vi "niFpgaFFTStreamingOutputControlUnit.vi"(0 "reset":bool, 5 "ready for output":bool, 7 "current status":enum8{"idle", "output"}(ring), 9 "execution constants":cluster{"bitmask":u16, "K-16":i8}={"bitmask"=2047, "K-16"=-5}) -> (4 "output valid (inside)":bool, 6 "next status":enum8{"idle", "output"}(ring), 8 "data index":u16, 10 "use buffer 0":bool, 13 "read address 1":u16, 14 "read address 0":u16)   [LabVIEW 2017]
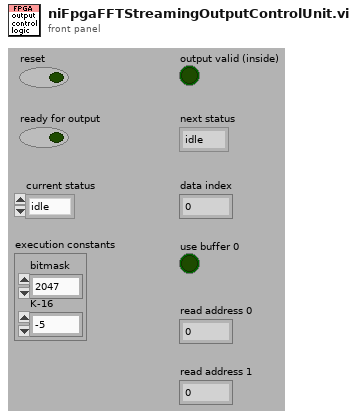
[diagram p1: front panel]
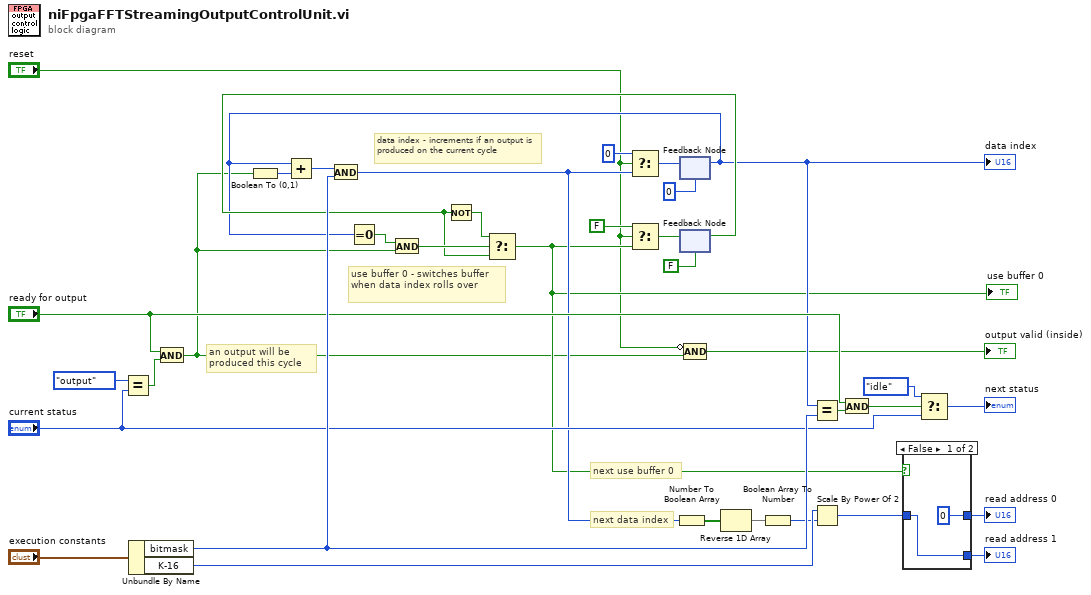
[diagram p0: block diagram]
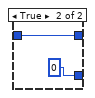
[diagram p2: hidden frame]
diagram:
  # "an output will be produced this cycle"
  # "use buffer 0 - switches buffer when data index rolls over"
  # "data index - increments if an output is produced on the current cycle"
  # "next data index"
  # "next use buffer 0"
  n1 = Equal?(x=enum8{"idle", "output"}."output" ("current status"), y="current status") -> (x = y?=w30:bool)
  n2 = Unbundle By Name("execution constants") -> ("bitmask"=w25:u16, "K-16"=w32:i8)
  n3 = And(x="ready for output", y=w30) -> (x .and. y?=w3:bool)
  n4 = Boolean To (0,1)(Boolean=w3) -> (0, 1=w22:i16)
  n5 = feedback #1(u16 0 ("t")) -> (w7:u16)
  "data index" <- w7
  n6 = Add(x=w7, y=w22) -> (x+y=w21:u16)
  n7 = And(x=w21, y=w25) -> (x .and. y?=w13:u16)
  n8 = Equal To 0?(x=w7) -> (x = 0?=w18:bool)
  n9 = And(x=w18, y=w3) -> (x .and. y?=w17:bool)
  n10 = Select(t=u16 0, s="reset", f=w13) -> (s? t:f=w11:u16)
  n11 = Number To Boolean Array(number=w13) -> (Boolean array=w35:bool[])
  n12 = feedback-in #1(w11) -> ()
  n13 = feedback #2(FALSE ("t")) -> (w8:bool)
  n14 = Not(x=w8) -> (.not. x?=w16:bool)
  n15 = Select(t=w16, s=w17, f=w8) -> (s? t:f=w5:bool)
  "use buffer 0" <- w5
  n16 = Select(t=FALSE, s="reset", f=w5) -> (s? t:f=w12:bool)
  n17 = feedback-in #2(w12) -> ()
  n18 = Compound Arithmetic op=AND(invert "reset", w3) -> (→"output valid (inside)":bool)
  n19 = Reverse 1D Array(array=w35) -> (reversed array=w34:bool[])
  n20 = Boolean Array To Number(Boolean array=w34) -> (number=w23:u16)
  n21 = Equal?(x=w7, y=w25) -> (x = y?=w15:bool)
  n22 = Scale By Power Of 2(n=w32, x=w23) -> (x*2^n=w24:u16)
  n23 = And(x="ready for output", y=w15) -> (x .and. y?=w29:bool)
  n24 = case shown="False" w5 {
    tunnel: w24 -> [w37 w39]
    tunnel: [u16 0 w39] -> w27
    tunnel: [w37 u16 0] -> w26
    frame False {
    }
    frame True {
    }
  }
  "read address 0" <- w27
  "read address 1" <- w26
  n25 = Select(t=enum8{"idle", "output"}."idle", s=w29, f="current status") -> (s? t:f=→"next status":enum8{"idle", "output"})
